vi "Get_Dll_Data.vi"(8 "error in (no error)":errorcluster, 11 "Class in":refnum<class "AB_DLL.lvclass">) -> (0 "error out":errorcluster, 2 "data":T1, 3 "Class out":refnum<class "AB_DLL.lvclass">)   [LabVIEW 2020, in "AB_DLL.lvclass"]
uses:
  <vilib>/AppBuilder/AB_Classes/DLL/AB_DLL.lvclass
  <vilib>/AppBuilder/AB_Classes/DLL/AB_DLL.ctl
  <vilib>/AppBuilder/AB_Classes/DLL/AB_DLL.lvclass/AB_DLL.ctl
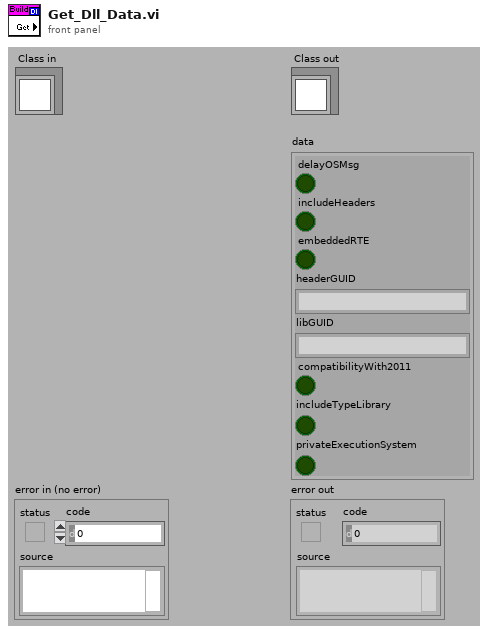
[diagram p1: front panel]
types:
  T1 = typedef "AB_DLL.ctl" = cluster{"delayOSMsg":bool, "includeHeaders":bool, "embeddedRTE":bool, "headerGUID":string, "libGUID":string, "compatibilityWith2011":bool, "includeTypeLibrary":bool, "privateExecutionSystem":bool}
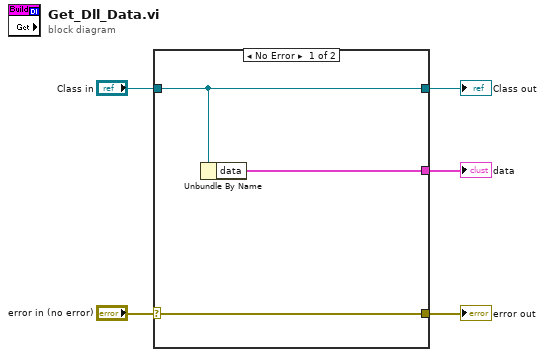
[diagram p0: block diagram]
diagram:
  n1 = case shown="No Error" "error in (no error)" {
    selector: "error in (no error)" -> [w8 w10]
    tunnel: [w8 w10] -> w4
    tunnel: [w7 w9] -> w2
    tunnel: "Class in" -> [w7 w9]
    tunnel: [w6 _] -> w1
    frame No Error {
      n2 = Unbundle By Name(w7) -> ("data"=w6:T1)
    }
    frame Error {
    }
  }
  "Class out" <- w2
  "error out" <- w4
  "data" <- w1
